vi "AddControlByPath__slk_mt.vi"(7 "position (0,0)":T1, 8 "error in (no error)":errorcluster, 10 "path":path, 11 "owner vi refnum in":refnum<vi>) -> (0 "error out":errorcluster, 3 "control refnum out":refnum<vi>)   [LabVIEW 2015, in "Lazyboots Menu Tool.lvlib"]
doc: "Adds control to the specified position by control path."
uses:
  <vilib>/SLK/Lazyboots Menu Tool/Library/Lazyboots Menu Tool.lvlib
  <vilib>/Utility/miscctls.llb/LVPositionTypeDef.ctl
  <vilib>/Utility/miscctls.llb/LVPointTypeDef.ctl
panel:
  # "AddControlByPath__slk_mt.vi\nAdds control to the specified position by control path.\n\nNOTICE -- YOU MUST LEAVE THIS NOTICE IN PLACE.\n\nCopyright (c) 2011, LIANG LIU Shawn.Liu.cn@gmail.com\nAll rights reserved.\n\nRedistribution and use in source and binary forms, with or without modification, are permitted provided that the following conditions are met:\n-Redistributions of source code must retain the above copyright notice, this list of conditions and the following disclaimer.\n-Redistributions in binary form must reproduce the above copyright notice, this list of conditions and the following disclaimer in the documentation and/or other materials provided with the distribution.\n-Neither the name of the eLp nor the names of its contributors may be used to endorse or promote products derived from this software without specific prior written permission.\n\nTHIS SOFTWARE IS PROVIDED BY THE COPYRIGHT HOLDERS AND CONTRIBUTORS \"AS IS\" AND ANY EXPRESS OR IMPLIED WARRANTIES, INCLUDING, BUT NOT LIMITED TO, THE IMPLIED WARRANTIES OF MERCHANTABILITY AND FITNESS FOR A PARTICULAR PURPOSE ARE DISCLAIMED. IN NO EVENT SHALL THE COPYRIGHT HOLDER OR CONTRIBUTORS BE LIABLE FOR ANY DIRECT, INDIRECT, INCIDENTAL, SPECIAL, EXEMPLARY, OR CONSEQUENTIAL DAMAGES (INCLUDING, BUT NOT LIMITED TO, PROCUREMENT OF SUBSTITUTE GOODS OR SERVICES; LOSS OF USE, DATA, OR PROFITS; OR BUSINESS INTERRUPTION) HOWEVER CAUSED AND ON ANY THEORY OF LIABILITY, WHETHER IN CONTRACT, STRICT LIABILITY, OR TORT (INCLUDING NEGLIGENCE OR OTHERWISE) ARISING IN ANY WAY OUT OF THE USE OF THIS SOFTWARE, EVEN IF ADVISED OF THE POSSIBILITY OF SUCH DAMAGE."
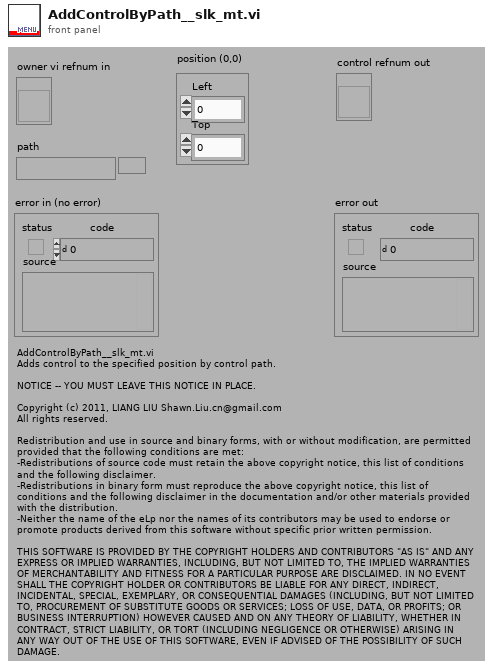
[diagram p1: front panel]
types:
  T1 = typedef "LVPositionTypeDef.ctl" = cluster{"Left":i32, "Top":i32}
  T2 = typedef "LVPointTypeDef.ctl" = cluster{"Horizontal":i16, "Vertical":i16}
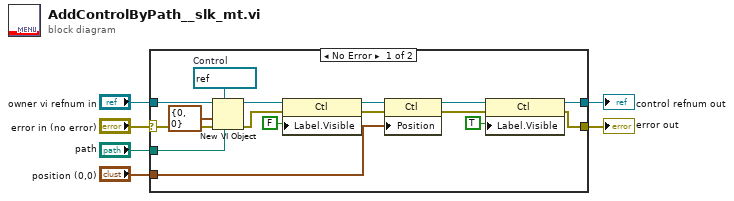
[diagram p0: block diagram]
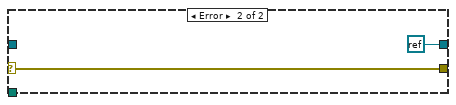
[diagram p2: hidden frame]
diagram:
  n1 = case shown="No Error" "error in (no error)" {
    selector: "error in (no error)" -> [w8 w24]
    tunnel: "position (0,0)" -> [w14 _]
    tunnel: "owner vi refnum in" -> [w12 _]
    tunnel: [w11 refnum<k0> refnum] -> w4
    tunnel: "path" -> [w10 _]
    tunnel: [w9 w24] -> w2
    frame No Error {
      w7 = refnum<vi> refnum  # Control
      n2 = New VI Object(vi object class=w7, owner refnum=w12, position/next to=T2 {"Horizontal"=0, "Vertical"=0} ("relative position/next to refnum"), 6:w10, 8:w8) -> (object refnum=w19:refnum<vi>, 0:w16:errorcluster)  [unwired: 1 in, 2 out]
      n3 = property class="Ctl"(reference=w19, error in=w16, "Label.Visible"=FALSE) -> (reference out=w20:refnum<vi>, error out=w22:errorcluster)
      n4 = property class="Ctl"(reference=w20, error in=w22, "Position"=w14) -> (reference out=w21:refnum<vi>, error out=w17:errorcluster)
      n5 = property class="Ctl"(reference=w21, error in=w17, "Label.Visible"=TRUE) -> (reference out=w11:refnum<vi>, error out=w9:errorcluster)
    }
    frame Error {
    }
  }
  "control refnum out" <- w4
  "error out" <- w2
